vi "StartCapture.vi"(8 "error in (no error)":errorcluster, 10 "Continuous":bool, 11 "Inovance_Camera in":refnum<class "Inovance_Camera.lvclass">) -> (0 "error out":errorcluster, 3 "Inovance_Camera out":refnum<class "Inovance_Camera.lvclass">)   [LabVIEW 2023, in "Inovance_Camera.lvlib" / "Inovance_Camera.lvclass"]
uses:
  Inovance_Camera.lvclass
  <vilib>/userDefined/High Color/IMAQdx.ctl
  <vilib>/ActorFramework/Actor/Actor.lvclass/Actor.ctl
  Inovance_Camera.lvclass/Inovance_Camera.ctl
  <vilib>/ActorFramework/Message Enqueuer/Message Enqueuer.lvclass/Message Enqueuer.ctl
  <vilib>/ActorFramework/Message Enqueuer/Enqueue.vi
  Interfaces/AbstractInstrumentClasses/Cameras_LV/CameraComm Messages/Capture Started Msg/Capture Started Msg.lvclass
  <vilib>/ActorFramework/Message Priority Queue/Priority Enqueue.vi
  <vilib>/vision/driver/NI_Vision_Acquisition_Software.lvlib
  <vilib>/ActorFramework/Actor/Actor.lvclass
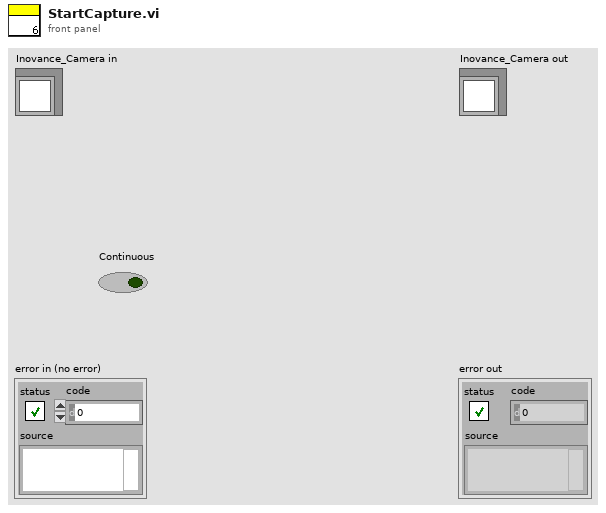
[diagram p1: front panel]
types:
  T1 = typedef "IMAQdx.ctl" = refnum<k21>
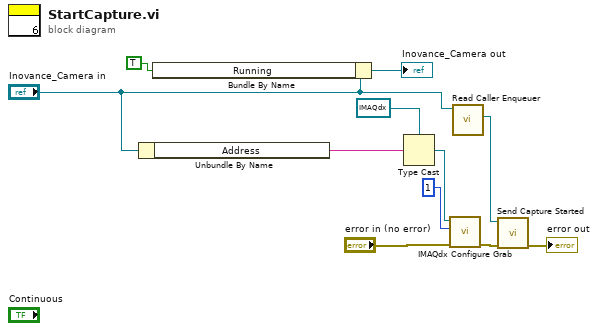
[diagram p0: block diagram]
diagram:
  n1 = Unbundle By Name("Inovance_Camera in") -> ("Address"=w6:string)
  n2 = Bundle By Name(cluster="Inovance_Camera in", "Running"=TRUE ("InstrumentData.CurrentState.Running")) -> (→"Inovance_Camera out":refnum<class "Inovance_Camera.lvclass">)
  n3 = Type Cast(type=T1 refnum ("Inovance Address"), x=w6) -> (*(type *) &x=w4:T1)
  n4 = call <vilib>:"IMAQdx Configure Grab.vi"("error in"="error in (no error)", "Number of Buffers"=u32 1, "Session In"=w4) -> ("error out"=w9:errorcluster)  [unwired: 7 in, 1 out]
  n5 = call <vilib>:"Read Caller Enqueuer.vi"("Actor"="Inovance_Camera in") -> ("Caller Enqueuer"=w7:refnum<class "Message Enqueuer.lvclass">)  [unwired: 10 in]
  n6 = call "Send Capture Started.vi"("error in (no error)"=w9, "Message Enqueuer"=w7) -> ("error out"=→"error out":errorcluster)  [unwired: 8 in, 1 out]
